vi "Close.vi"(8 "error in (no error)":errorcluster, 11 "AbstractBattery in":refnum<class "AbstractBattery.lvclass">) -> (0 "error out":errorcluster, 3 "AbstractBattery out":refnum<class "AbstractBattery.lvclass">)   [LabVIEW 2013, in "AbstractBattery.lvclass"]
uses:
  AbstractBattery.lvclass
  AbstractBattery.lvclass/AbstractBattery.ctl
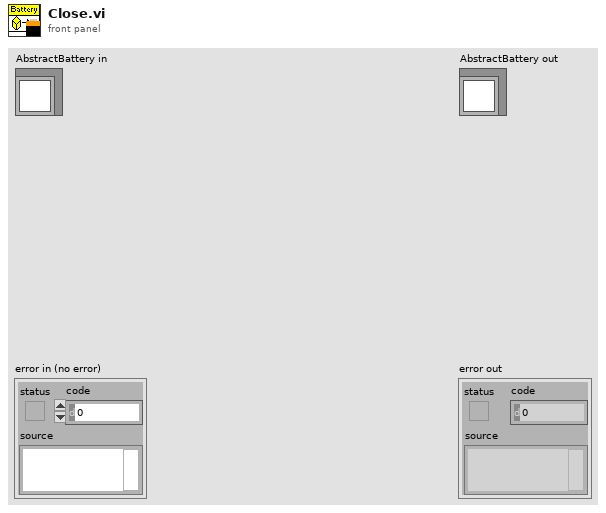
[diagram p1: front panel]
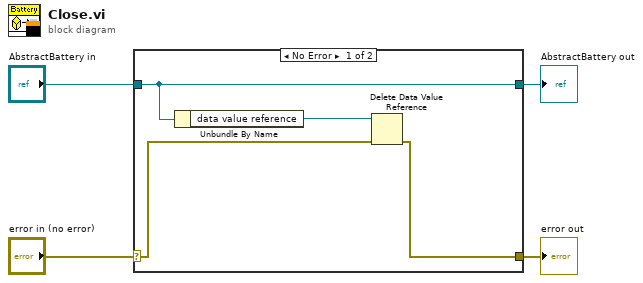
[diagram p0: block diagram]
diagram:
  n1 = case shown="No Error" "error in (no error)" {
    selector: "error in (no error)" -> [w7 w9]
    tunnel: [w6 w9] -> w3
    tunnel: [w5 w10] -> w1
    tunnel: "AbstractBattery in" -> [w5 w10]
    frame No Error {
      n2 = Unbundle By Name(w5) -> ("data value reference"=w8:refnum<data-value>)
      n3 = Delete Data Value Reference(data value reference=w8, error in=w7) -> (error out=w6:errorcluster)  [unwired: 1 out]
    }
    frame Error {
    }
  }
  "error out" <- w3
  "AbstractBattery out" <- w1
